vi "non_linear_fitting_subvi.vi"(6 "Fitting Function":string, 7 "Parameter array":T1(array[cluster]), 8 "error in (no error)":errorcluster, 9 "termination":cluster{"max iteration":i32, "tolerance":dbl}, 10 "Y":dbl[](array[numeric]), 11 "X":dbl[](array[numeric])) -> (0 "error out":errorcluster, 1 "best fit parameter":dbl[](array[numeric]), 2 "XY graph out (original + fit)":cluster{"X":dbl[], "best nonlinear fit":dbl[]}[](array[cluster]), 3 "best nonlinear fit":dbl[](array[numeric]))   [LabVIEW 2025]
uses:
  <vilib>/gmath/NumericalOptimization/Nonlinear Curve Fit LM formula string.vi
  <vilib>/gmath/NI_Gmath.lvlib
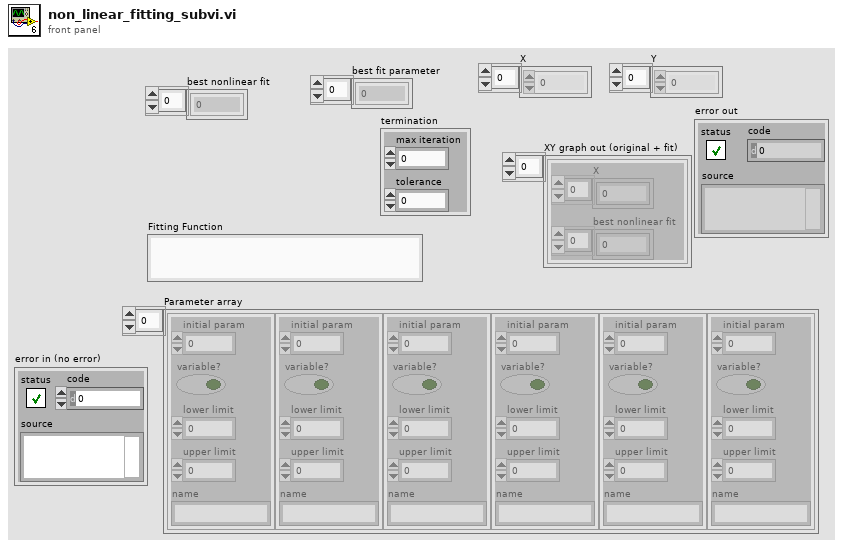
[diagram p1: front panel]
types:
  T1 = cluster{"initial param":dbl, "variable?":bool, "lower limit":dbl, "upper limit":dbl, "name":string}[]
  T2 = cluster{"model":string, "Parameters":string[], "x":string}
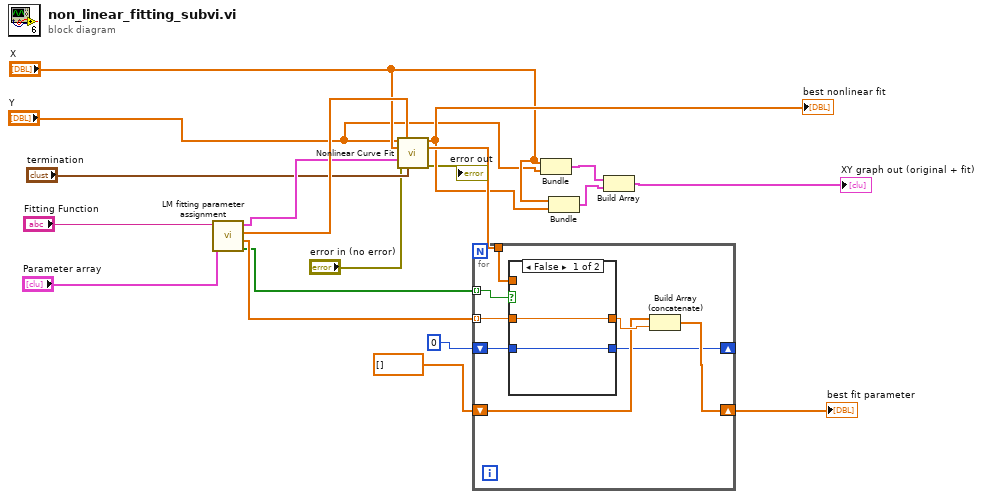
[diagram p0: block diagram]
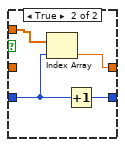
[diagram p2: hidden frame]
diagram:
  n1 = call "LM fitting parameter assignment.vi"("Parameter array"="Parameter array", "Fitting Function (write with ai's)"="Fitting Function") -> ("boolean array"=w14:bool[], "initial initial"=w15:dbl[], "initial parameters"=w13:dbl[], "Output for LM fitting"=w5:T2)  [unwired: 6 in]
  n2 = call-poly <vilib>:"Nonlinear Curve Fit.vi"("Y"="Y", "initial parameters"=w13, "X"="X", "model description"=w5, "error in (no error)"="error in (no error)", "termination"="termination") -> ("best nonlinear fit"=w10:dbl[], "best fit parameters"=w17:dbl[], "error out"=→"error out":errorcluster)  [unwired: 5 in, 2 out]
  "best nonlinear fit" <- w10
  n3 = for {
    tunnel: w14 -> [w27] mode=indexing
    tunnel: w15 -> [w25] mode=indexing
    shift-right: [w23] -> w19
    shift-left: dbl[] [] ("appended array") -> [w24]
    tunnel: w17 -> [w22]
    shift-right: [w21] -> _
    shift-left: 0 -> [w20]
    n4 = case shown="False" w27 {
      tunnel: [w28 w30] -> w26
      tunnel: w25 -> [w28 _]
      tunnel: w22 -> [_ w32]
      tunnel: [w29 w33] -> w21
      tunnel: w20 -> [w29 w31]
      frame False {
      }
      frame True {
        n5 = Index Array(array=w32, index=w31) -> (element=w30:dbl)
        n6 = Increment(x=w31) -> (x+1=w33:i32)
      }
    }
    n7 = Build Array (concatenate)(w24, w26) -> (w23:dbl[])
  }
  "best fit parameter" <- w19
  n8 = Bundle("X"="X", "Y"="Y") -> (w7:cluster{"X":dbl[], "Y":dbl[]})  [unwired: 1 in]
  n9 = Bundle("X"="X", "best nonlinear fit"=w10) -> (w11:cluster{"X":dbl[], "best nonlinear fit":dbl[]})  [unwired: 1 in]
  n10 = Build Array(w7, w11) -> (→"XY graph out (original + fit)":cluster{"X":dbl[], "best nonlinear fit":dbl[]}[])
